vi "NPRManager.vi"(3 "error in (no error)":errorcluster caption="错误输入（无错误）", 4 "Input":T2, 5 "ref_in":T1) -> (0 "error out":errorcluster caption="错误输出", 1 "Output":T2, 2 "ref_out":T1)   [LabVIEW 2012]
uses:
  D:/workspace/GitHub/LVsolis/lib/AgilisCmdLib.dll
  lib/AgilisCmdLib.dll
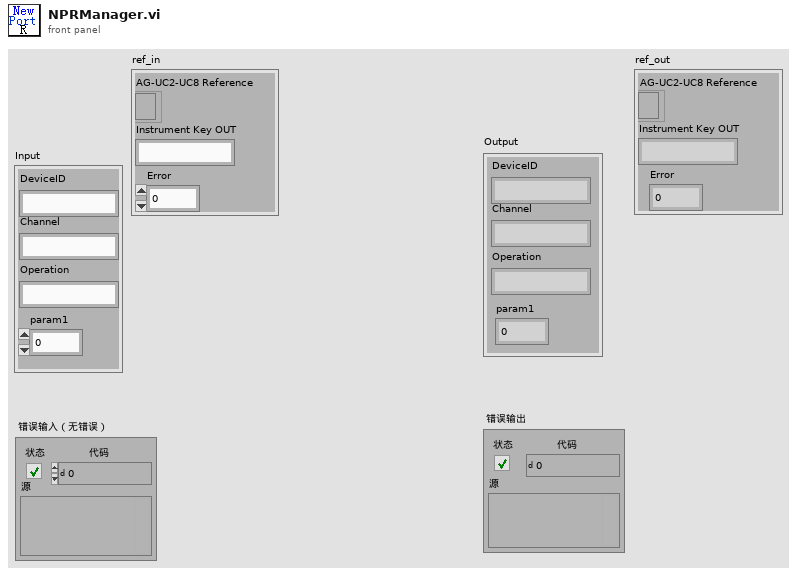
[diagram p1: front panel]
types:
  T1 = cluster{"AG-UC2-UC8 Reference":refnum<k24>, "Instrument Key OUT":string, "Error":i32}
  T2 = cluster{"DeviceID":string, "Channel":string, "param1":dbl, "Operation":string}
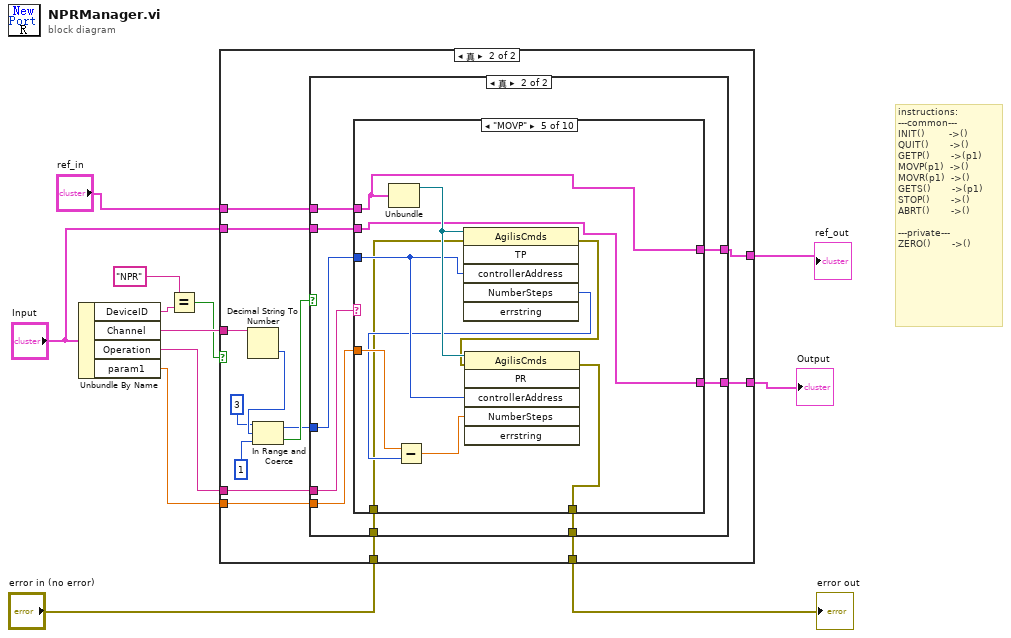
[diagram p0: block diagram]
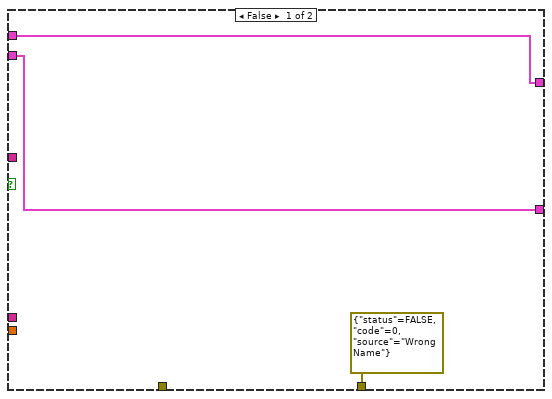
[diagram p2: hidden frame]
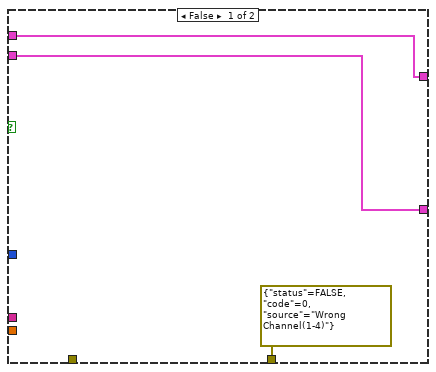
[diagram p3: hidden frame]
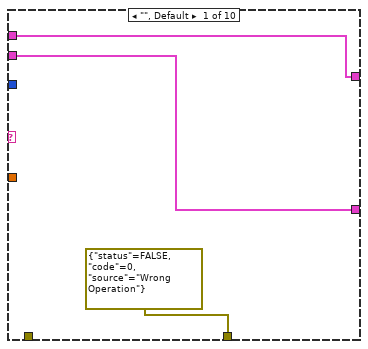
[diagram p4: hidden frame]
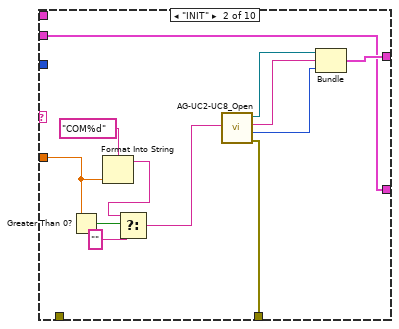
[diagram p5: hidden frame]
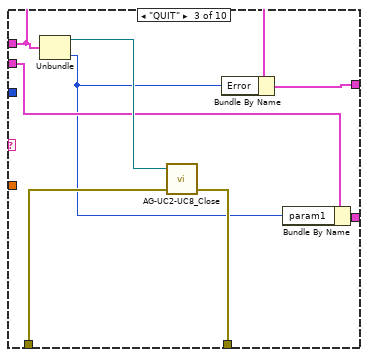
[diagram p6: hidden frame]
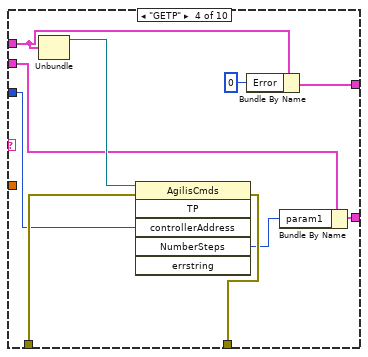
[diagram p7: hidden frame]
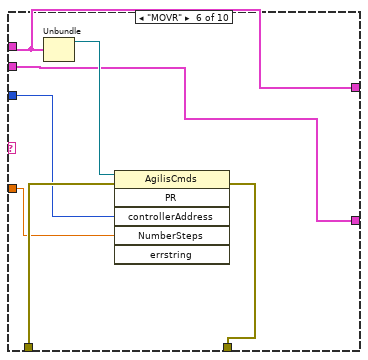
[diagram p8: hidden frame]
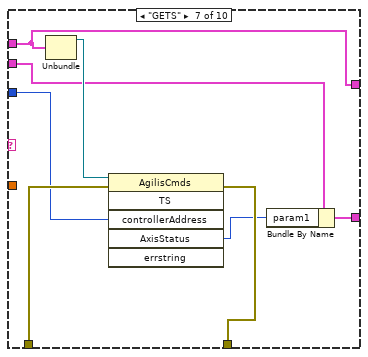
[diagram p9: hidden frame]
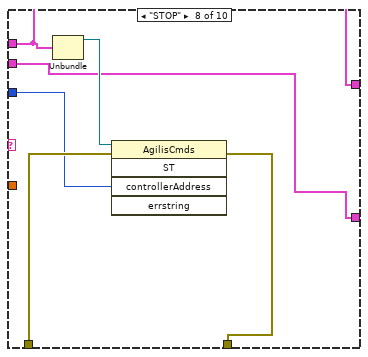
[diagram p10: hidden frame]
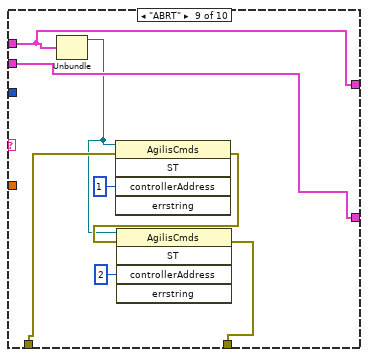
[diagram p11: hidden frame]
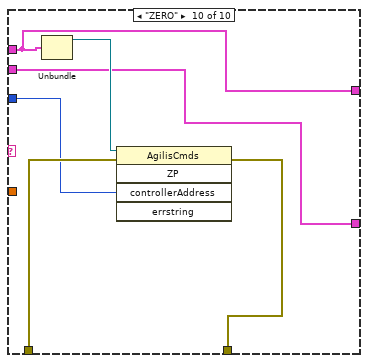
[diagram p12: hidden frame]
diagram:
  # "instructions:\n---common---\nINIT()        ->()\nQUIT()       ->()\nGETP()       ->(p1)\nMOVP(p1)  ->()\nMOVR(p1)  ->()\nGETS()       ->(p1)\nSTOP()       ->()\nABRT()       ->()\n\n---private---\nZERO()       ->()"
  n1 = Unbundle By Name("Input") -> ("DeviceID"=w12:string, "Channel"=w10:string, "Operation"=w9:string, "param1"=w8:dbl)
  n2 = Equal?(x="NPR", y=w12) -> (x = y?=w3:bool)
  n3 = case shown="真" w3 {
    tunnel: w10 -> [_ w29]
    tunnel: w9 -> [_ w23]
    tunnel: w8 -> [_ w22]
    tunnel: "error in (no error)" -> [_ w21]
    tunnel: [errorcluster {"status"=FALSE, "code"=0, "source"="Wrong Name"} ("error out") w20] -> w6
    tunnel: [w15 w19] -> w5
    tunnel: "ref_in" -> [w13 w18]
    tunnel: "Input" -> [w15 w17]
    tunnel: [w13 w16] -> w2
    frame False {
    }
    frame True {
      n4 = Decimal String To Number(string=w29) -> (number=w28:i32)  [unwired: 2 in, 1 out]
      n5 = In Range and Coerce(upper limit=3 ("上限"), x=w28, lower limit=1 ("下限")) -> (coerced(x)=w24:i32, In Range?=w25:bool)
      n6 = case shown="真" w25 {
        tunnel: w24 -> [_ w40]
        tunnel: w23 -> [_ w41]
        tunnel: w22 -> [_ w39]
        tunnel: w21 -> [_ w38]
        tunnel: [errorcluster {"status"=FALSE, "code"=0, "source"="Wrong Channel(1-4)"} ("error out") w37] -> w20
        tunnel: [w32 w36] -> w19
        tunnel: w18 -> [w30 w35]
        tunnel: w17 -> [w32 w34]
        tunnel: [w30 w33] -> w16
        frame False {
        }
        frame True {
          n7 = case shown="\"MOVP\"" w41 {
            tunnel: w40 -> [_ _ _ w65 w83 w88 w96 w102 _ w116]
            tunnel: w39 -> [_ w54 _ _ w81 w87 _ _ _ _]
            tunnel: w38 -> [_ _ w63 w74 w77 w90 w98 w104 w112 w118]
            tunnel: [errorcluster {"status"=FALSE, "code"=0, "source"="Wrong Operation"} ("error out") w47 w62 w73 w75 w89 w97 w103 w109 w117] -> w37
            tunnel: [w44 w45 w59 w70 w78 w85 w95 w101 w113 w114] -> w36
            tunnel: w35 -> [w42 _ w60 w68 w79 w86 w92 w100 w106 w115]
            tunnel: w34 -> [w44 w45 w58 w69 w78 w85 w94 w101 w113 w114]
            tunnel: [w42 w48 w61 w71 w79 w86 w92 w100 w106 w115] -> w33
            frame "", Default {
            }
            frame "INIT" {
              n8 = Greater Than 0?(x=w54) -> (x > 0?=w56:bool)
              n9 = Format Into String(format string="COM%d" ("格式字符串"), w54) -> (resulting string=w53:string)  [unwired: 2 in, 1 out]
              n10 = Select(t=w53, s=w56, f="") -> (s? t:f=w51:string)
              n11 = call "AG-UC2-UC8_Open.vi"("Instrument Key IN"=w51) -> ("error out"=w47:errorcluster, "Error"=w46:i32, "Instrument Key OUT"=w49:string, "AG-UC2-UC8 Reference"=w50:refnum<k24>)  [unwired: 3 in]
              n12 = Bundle("AG-UC2-UC8 Reference"=w50, "Instrument Key OUT"=w49, "Error"=w46) -> (w48:T1)  [unwired: 1 in]
            }
            frame "QUIT" {
              n13 = Unbundle(w60) -> ("AG-UC2-UC8 Reference"=w64:refnum<k24>, "Error"=w57:i32)  [unwired: 1 out]
              n14 = call "AG-UC2-UC8_Close.vi"("error in (no error)"=w63, "AG-UC2-UC8 Reference"=w64) -> ("Error out"=w62:errorcluster)  [unwired: 2 in, 1 out]
              n15 = Bundle By Name(cluster=w60, "Error"=w57) -> (w61:T1)
              n16 = Bundle By Name(cluster=w58, "param1"=w57) -> (w59:T2)
            }
            frame "GETP" {
              n17 = Unbundle(w68) -> ("AG-UC2-UC8 Reference"=w72:refnum<k24>)  [unwired: 2 out]
              n18 = invoke class="AgilisCmds" method="TP"(reference=w72, error in=w74, "controllerAddress"=w65) -> (error out=w73:errorcluster, "NumberSteps"=w67:i32)  [unwired: 3 in, 4 out]
              n19 = Bundle By Name(cluster=w68, "Error"=0) -> (w71:T1)
              n20 = Bundle By Name(cluster=w69, "param1"=w67) -> (w70:T2)
            }
            frame "MOVP" {
              n21 = Unbundle(w79) -> ("AG-UC2-UC8 Reference"=w84:refnum<k24>)  [unwired: 2 out]
              n22 = invoke class="AgilisCmds" method="TP"(reference=w84, error in=w77, "controllerAddress"=w83) -> (error out=w76:errorcluster, "NumberSteps"=w80:i32)  [unwired: 3 in, 4 out]
              n23 = Subtract(x=w81, y=w80) -> (x-y=w82:dbl)
              n24 = invoke class="AgilisCmds" method="PR"(reference=w84, error in=w76, "controllerAddress"=w83, "NumberSteps"=w82) -> (error out=w75:errorcluster)  [unwired: 2 in, 5 out]
            }
            frame "MOVR" {
              n25 = Unbundle(w86) -> ("AG-UC2-UC8 Reference"=w91:refnum<k24>)  [unwired: 2 out]
              n26 = invoke class="AgilisCmds" method="PR"(reference=w91, error in=w90, "controllerAddress"=w88, "NumberSteps"=w87) -> (error out=w89:errorcluster)  [unwired: 2 in, 5 out]
            }
            frame "GETS" {
              n27 = Unbundle(w92) -> ("AG-UC2-UC8 Reference"=w99:refnum<k24>)  [unwired: 2 out]
              n28 = invoke class="AgilisCmds" method="TS"(reference=w99, error in=w98, "controllerAddress"=w96) -> (error out=w97:errorcluster, "AxisStatus"=w93:i32)  [unwired: 3 in, 4 out]
              n29 = Bundle By Name(cluster=w94, "param1"=w93) -> (w95:T2)
            }
            frame "STOP" {
              n30 = Unbundle(w100) -> ("AG-UC2-UC8 Reference"=w105:refnum<k24>)  [unwired: 2 out]
              n31 = invoke class="AgilisCmds" method="ST"(reference=w105, error in=w104, "controllerAddress"=w102) -> (error out=w103:errorcluster)  [unwired: 2 in, 4 out]
            }
            frame "ABRT" {
              n32 = Unbundle(w106) -> ("AG-UC2-UC8 Reference"=w108:refnum<k24>)  [unwired: 2 out]
              n33 = invoke class="AgilisCmds" method="ST"(reference=w108, error in=w112, "controllerAddress"=1) -> (error out=w110:errorcluster)  [unwired: 2 in, 4 out]
              n34 = invoke class="AgilisCmds" method="ST"(reference=w108, error in=w110, "controllerAddress"=2) -> (error out=w109:errorcluster)  [unwired: 2 in, 4 out]
            }
            frame "ZERO" {
              n35 = Unbundle(w115) -> ("AG-UC2-UC8 Reference"=w119:refnum<k24>)  [unwired: 2 out]
              n36 = invoke class="AgilisCmds" method="ZP"(reference=w119, error in=w118, "controllerAddress"=w116) -> (error out=w117:errorcluster)  [unwired: 2 in, 4 out]
            }
          }
        }
      }
    }
  }
  "Output" <- w5
  "error out" <- w6
  "ref_out" <- w2
